vi "make_DMD.vi"() -> ()   [LabVIEW 2012]
panel:
  out "Image":dbl[][](graph)
  out "Real":dbl
  in  "Numeric":dbl
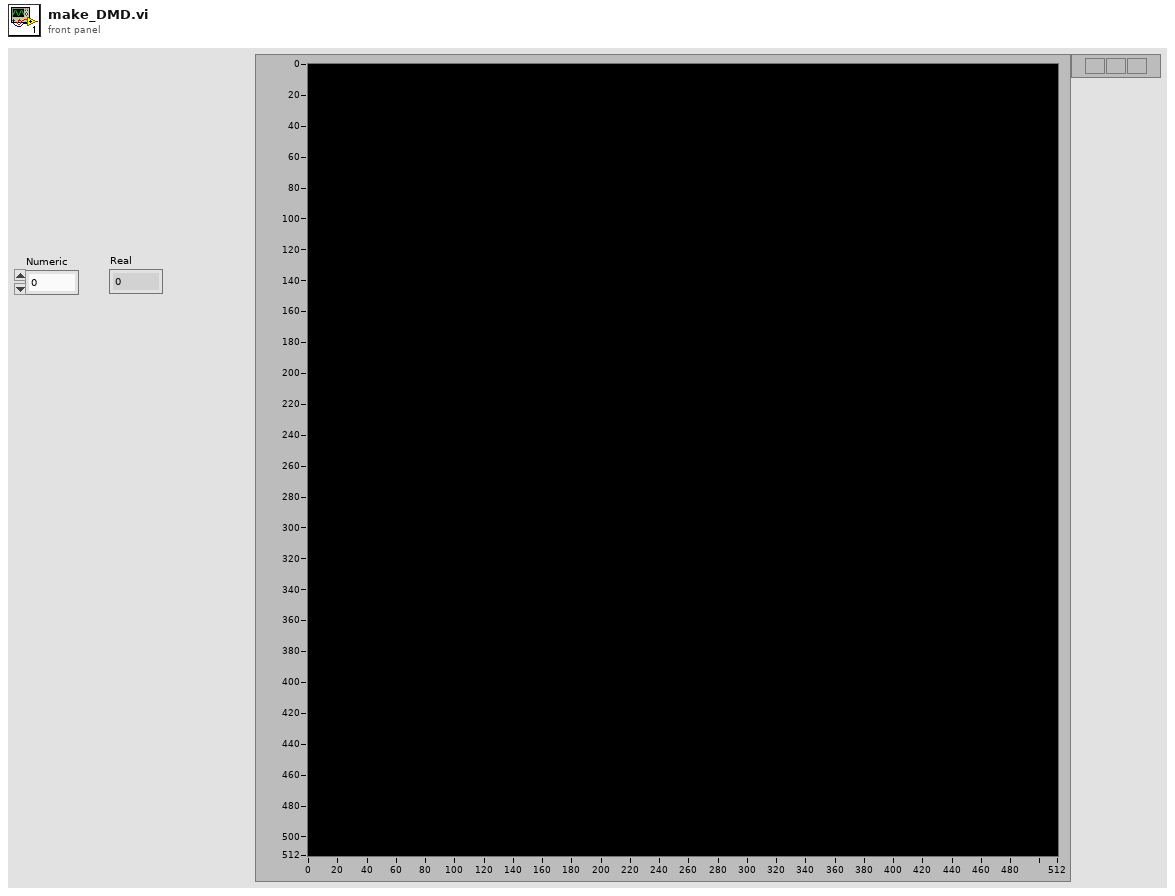
[diagram p1: front panel]
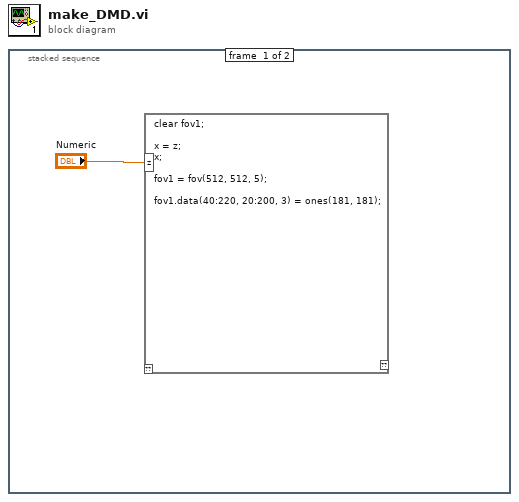
[diagram p0: block diagram]
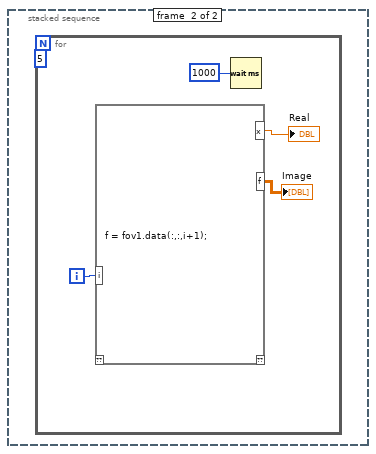
[diagram p2: hidden frame]
diagram:
  n1 = stacked-sequence {
    frame #0 {
      n2 = script code="clear fov1; \n\nx = z; \nx;  \n\nfov1 = fov(512, 512, 5); \n\nfov1.data(40:220, 20:200, 3) = ones(181, 181);"("z"="Numeric") -> ()  [unwired: 1 in, 1 out]
    }
    frame #1 {
      n3 = for {
        N: 5 -> [_]
        i -> [w6]
        n4 = script code="f = fov1.data(:,:,i+1);"("i"=w6) -> ("x"=→"Real":dbl, "f"=→"Image":dbl[][])  [unwired: 1 in, 1 out]
        n5 = Wait (ms)(milliseconds to wait=1000) -> ()  [unwired: 1 out]
      }
    }
  }
